vi "ParamParser.vi"(10 "Path":path) -> (0 "Calib File Selected?":bool, 2 "Calibration values":string[][](array[string]))   [LabVIEW 2010]
uses:
  <vilib>/Utility/file.llb/Read From Spreadsheet File (string).vi
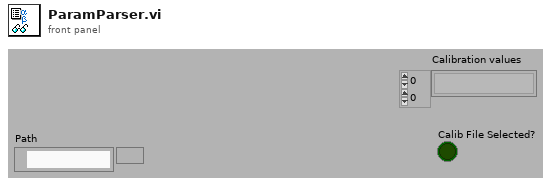
[diagram p1: front panel]
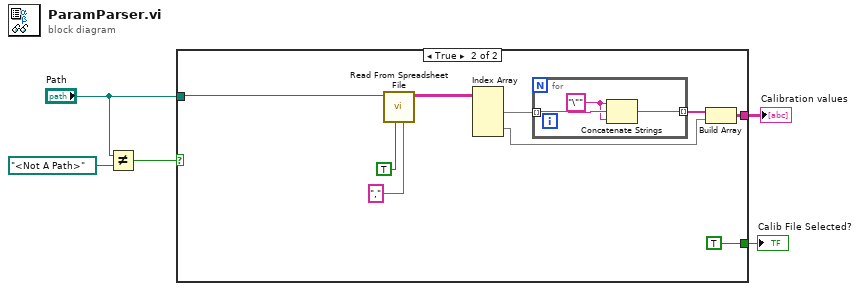
[diagram p0: block diagram]
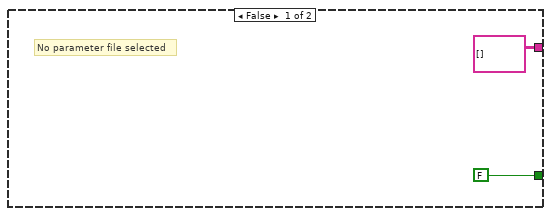
[diagram p2: hidden frame]
diagram:
  n1 = Not Equal?(x="Path", y=path "<Not A Path>") -> (x != y?=w4:bool)
  n2 = case shown="True" w4 {
    tunnel: [string[][] [] w10] -> w5
    tunnel: "Path" -> [_ w8]
    tunnel: [FALSE TRUE] -> w2
    frame False {
      # "No parameter file selected"
    }
    frame True {
      n3 = call-poly <vilib>:"Read From Spreadsheet File.vi"("delimiter (\\t)"="," ("delimiter (\\t)"), "transpose (no:F)"=TRUE, "file path (dialog if empty)"=w8) -> ("all rows"=w14:string[][])  [unwired: 4 in, 4 out]
      n4 = Index Array(array=w14) -> (element #1=w13:string[], element #2=w11:string[])  [unwired: 4 in]
      n5 = for {
        tunnel: w13 -> [w19] mode=indexing
        tunnel: [w17] -> w12 mode=indexing
        w18 = "\""
        n6 = Concatenate Strings(w18, w19, w18) -> (w17:string)
      }
      n7 = Build Array(w12, w11) -> (w10:string[][])
    }
  }
  "Calibration values" <- w5
  "Calib File Selected?" <- w2
